vi "DoorLock.vi"() -> ()   [LabVIEW 2017]
doc: "The myRIO Project template acquires acceleration data from the onboard accelerometer and displays the changes of acceleration values in a waveform chart."
uses:
  Button States Numlock.ctl
panel:
  out "Passcode (4 Digits)":string
  out "Wrong":bool
  out "Correct":bool
  in  "0":bool
  in  "3":bool
  in  "2":bool
  in  "1":bool
  in  "4":bool
  in  "5":bool
  in  "6":bool
  in  "9":bool
  in  "8":bool
  in  "7":bool
  in  "Enter Button":bool
  # "7"
  # "8"
  # "9"
  # "4"
  # "5"
  # "6"
  # "1"
  # "2"
  # "3"
  # "0"
  # "Status:"
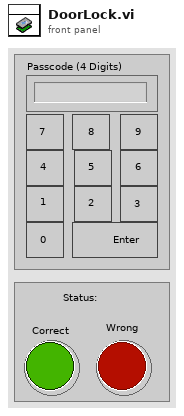
[diagram p1: front panel]
types:
  T1 = typedef "Button States Numlock.ctl" = enum16{"Wait", "0", "1", "2", "3", "4", "5", "6", "7", "8", "9", "Compare", "Wrong", "Correct"}
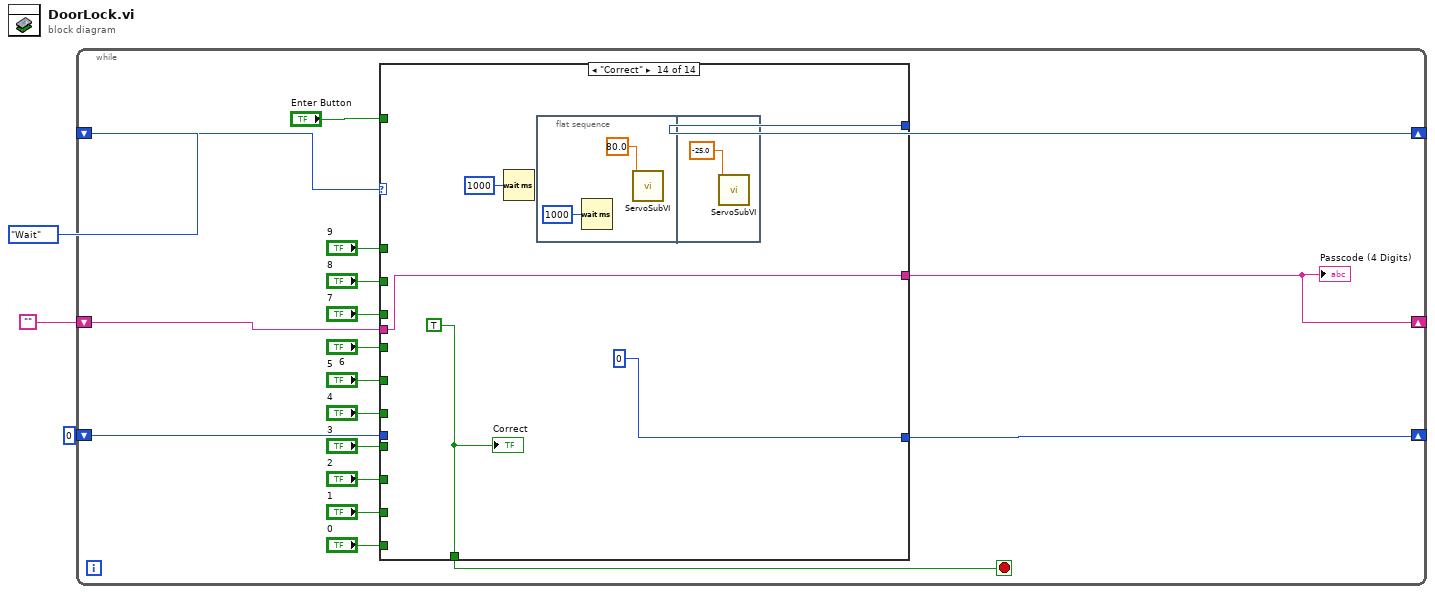
[diagram p0: block diagram]
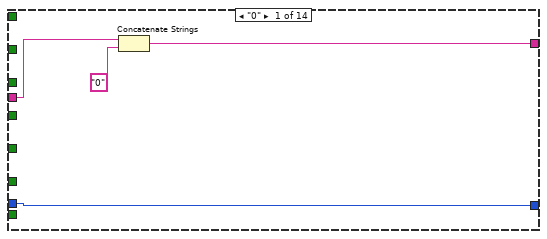
[diagram p2: hidden frame]
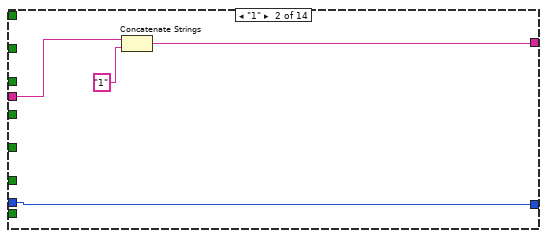
[diagram p3: hidden frame]
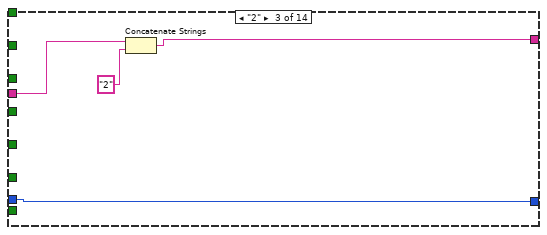
[diagram p4: hidden frame]
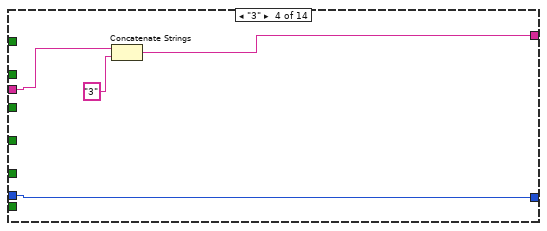
[diagram p5: hidden frame]
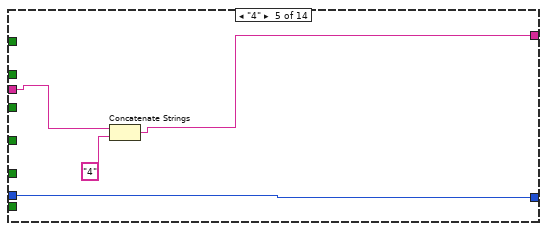
[diagram p6: hidden frame]
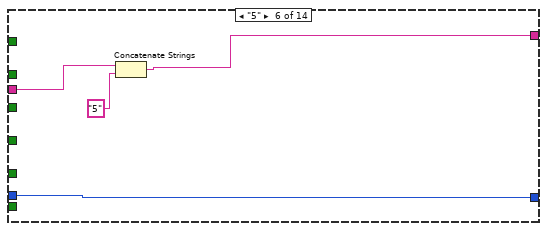
[diagram p7: hidden frame]
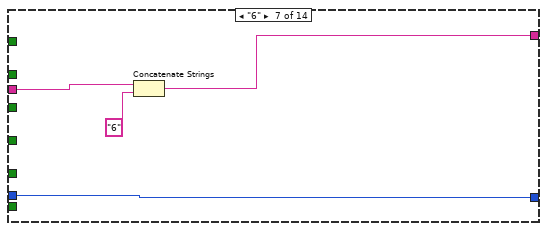
[diagram p8: hidden frame]
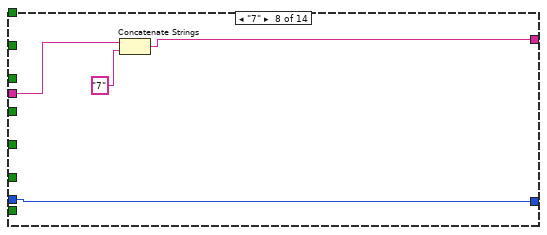
[diagram p9: hidden frame]
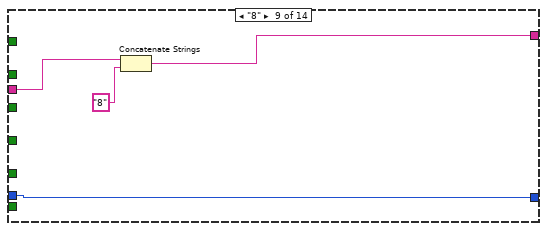
[diagram p10: hidden frame]
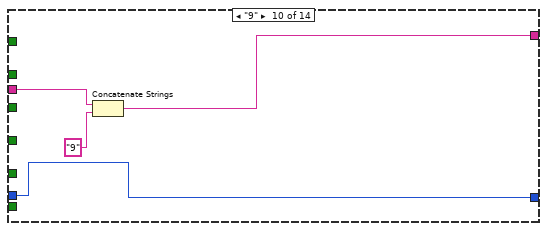
[diagram p11: hidden frame]
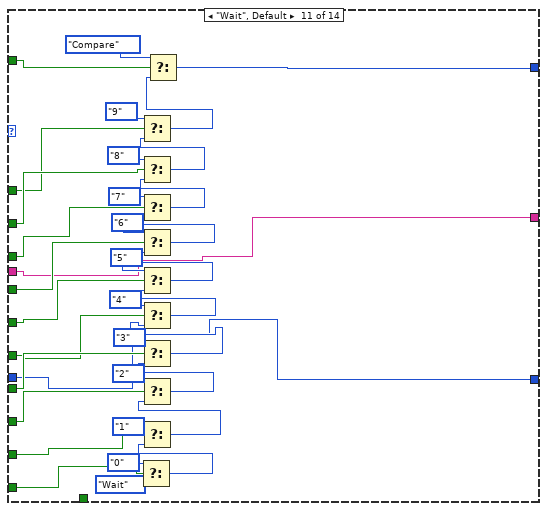
[diagram p12: hidden frame]
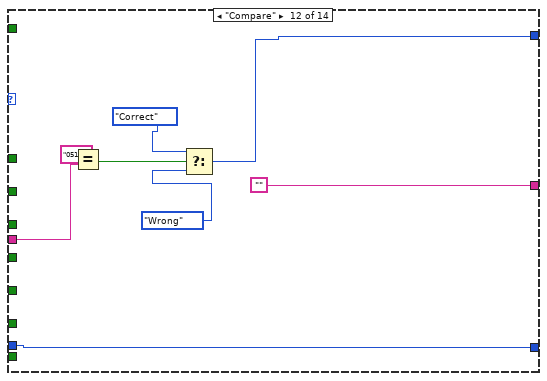
[diagram p13: hidden frame]
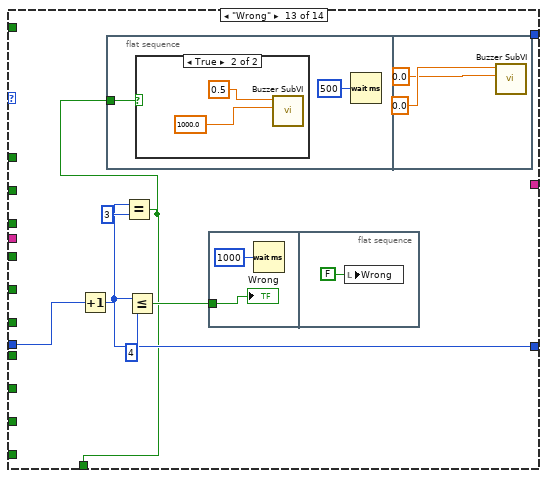
[diagram p14: hidden frame]
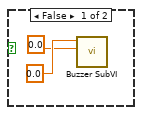
[diagram p15: hidden frame]
diagram:
  n1 = while {
    shift-right: [w7] -> _
    shift-left: Button_States_Numlock."Wait" -> [w11]
    shift-right: [w9] -> _
    shift-left: "" -> [w10]
    shift-right: [w5] -> _
    shift-left: 0 -> [w6]
    stop <- w4 stop-if-true
    n2 = case shown="\"Correct\"" w11 {
      tunnel: "0" -> [_ _ _ _ _ _ _ _ _ _ w95 _ _ _]
      tunnel: "1" -> [_ _ _ _ _ _ _ _ _ _ w80 _ _ _]
      tunnel: "2" -> [_ _ _ _ _ _ _ _ _ _ w79 _ _ _]
      tunnel: "4" -> [_ _ _ _ _ _ _ _ _ _ w77 _ _ _]
      tunnel: "3" -> [_ _ _ _ _ _ _ _ _ _ w78 _ _ _]
      tunnel: "5" -> [_ _ _ _ _ _ _ _ _ _ w76 _ _ _]
      tunnel: "6" -> [_ _ _ _ _ _ _ _ _ _ w75 _ _ _]
      tunnel: "7" -> [_ _ _ _ _ _ _ _ _ _ w74 _ _ _]
      tunnel: "8" -> [_ _ _ _ _ _ _ _ _ _ w69 _ _ _]
      tunnel: "9" -> [_ _ _ _ _ _ _ _ _ _ w68 _ _ _]
      tunnel: w10 -> [w25 w27 w31 w35 w39 w43 w47 w51 w55 w59 w67 w105 _ w126]
      tunnel: [w23 w28 w32 w36 w40 w44 w48 w52 w56 w60 w67 "" _ w126] -> w9
      tunnel: "Enter Button" -> [_ _ _ _ _ _ _ _ _ _ w66 _ _ _]
      tunnel: [_ _ _ _ _ _ _ _ _ _ w63 w100 _ _] -> w7
      tunnel: w6 -> [w22 w26 w30 w34 w38 w42 w46 w50 w54 w58 w62 w98 w111 _]
      tunnel: [w22 w26 w30 w34 w38 w42 w46 w50 w54 w58 w62 w98 w108 0] -> w5
      tunnel: [_ _ _ _ _ _ _ _ _ _ _ _ w106 w123] -> w4
      frame "0" {
        n3 = Concatenate Strings(w25, "0") -> (w23:string)
      }
      frame "1" {
        n4 = Concatenate Strings(w27, "1") -> (w28:string)
      }
      frame "2" {
        n5 = Concatenate Strings(w31, "2") -> (w32:string)
      }
      frame "3" {
        n6 = Concatenate Strings(w35, "3") -> (w36:string)
      }
      frame "4" {
        n7 = Concatenate Strings(w39, "4") -> (w40:string)
      }
      frame "5" {
        n8 = Concatenate Strings(w43, "5") -> (w44:string)
      }
      frame "6" {
        n9 = Concatenate Strings(w47, "6") -> (w48:string)
      }
      frame "7" {
        n10 = Concatenate Strings(w51, "7") -> (w52:string)
      }
      frame "8" {
        n11 = Concatenate Strings(w55, "8") -> (w56:string)
      }
      frame "9" {
        n12 = Concatenate Strings(w59, "9") -> (w60:string)
      }
      frame "Wait", Default {
        n13 = Select(t=Button_States_Numlock."0", s=w95, f=Button_States_Numlock."Wait") -> (s? t:f=w94:T1)
        n14 = Select(t=Button_States_Numlock."1", s=w80, f=w94) -> (s? t:f=w93:T1)
        n15 = Select(t=Button_States_Numlock."2", s=w79, f=w93) -> (s? t:f=w92:T1)
        n16 = Select(t=Button_States_Numlock."3", s=w78, f=w92) -> (s? t:f=w91:T1)
        n17 = Select(t=Button_States_Numlock."4", s=w77, f=w91) -> (s? t:f=w90:T1)
        n18 = Select(t=Button_States_Numlock."5", s=w76, f=w90) -> (s? t:f=w89:T1)
        n19 = Select(t=Button_States_Numlock."6", s=w75, f=w89) -> (s? t:f=w88:T1)
        n20 = Select(t=Button_States_Numlock."7", s=w74, f=w88) -> (s? t:f=w73:T1)
        n21 = Select(t=Button_States_Numlock."8", s=w69, f=w73) -> (s? t:f=w72:T1)
        n22 = Select(t=Button_States_Numlock."9", s=w68, f=w72) -> (s? t:f=w65:T1)
        n23 = Select(t=Button_States_Numlock."Compare", s=w66, f=w65) -> (s? t:f=w63:T1)
      }
      frame "Compare" {
        n24 = Equal?(x="0518", y=w105) -> (x = y?=w103:bool)
        n25 = Select(t=Button_States_Numlock."Correct", s=w103, f=Button_States_Numlock."Wrong") -> (s? t:f=w100:T1)
      }
      frame "Wrong" {
        n26 = Increment(x=w111) -> (x+1=w108:i32)
        n27 = flat-sequence {
          tunnel: w106 -> [w113]
          frame #0 {
            n28 = case shown="True" w113 {
              frame False {
                n29 = call "Buzzer SubVI.vi"("frequency [Hz]"=0.0, "Duty Cycle (0-1)"=0.0) -> ()  [unwired: 10 in]
              }
              frame True {
                n30 = call "Buzzer SubVI.vi"("frequency [Hz]"=1000.0, "Duty Cycle (0-1)"=0.5) -> ()  [unwired: 10 in]
              }
            }
            n31 = Wait (ms)(milliseconds to wait=u32 500) -> ()  [unwired: 1 out]
          }
          frame #1 {
            n32 = call "Buzzer SubVI.vi"("frequency [Hz]"=0.0, "Duty Cycle (0-1)"=0.0) -> ()  [unwired: 10 in]
          }
        }
        n33 = Equal?(x=w108, y=3) -> (x = y?=w106:bool)
        n34 = Less Or Equal?(x=w108, y=4) -> (x <= y?=w107:bool)
        n35 = flat-sequence {
          tunnel: w107 -> [w121]
          frame #0 {
            n36 = Wait (ms)(milliseconds to wait=u32 1000) -> ()  [unwired: 1 out]
            "Wrong" <- w121
          }
          frame #1 {
            n37 = local write "Wrong"(FALSE ("Wrong")) -> ()
          }
        }
      }
      frame "Correct" {
        w123 = TRUE
        n38 = Wait (ms)(milliseconds to wait=u32 1000) -> ()  [unwired: 1 out]
        n39 = flat-sequence {
          frame #0 {
            n40 = Wait (ms)(milliseconds to wait=u32 1000) -> ()  [unwired: 1 out]
            n41 = call "ServoSubVI.vi"("x"=80.0) -> ()  [unwired: 11 in]
          }
          frame #1 {
            n42 = call "ServoSubVI.vi"("x"=-25.0) -> ()  [unwired: 11 in]
          }
        }
        "Correct" <- w123
      }
    }
    "Passcode (4 Digits)" <- w9
  }
